vi "FindMaxnIndex.vi"() -> (1 "Numeric":i32, 3 "String":string)   [LabVIEW 2020]
uses:
  <vilib>/Utility/file.llb/Read Delimited Spreadsheet (string).vi
panel:
  out "number":i32[][](array[numeric])
  out "all rows":string[][](array[string])
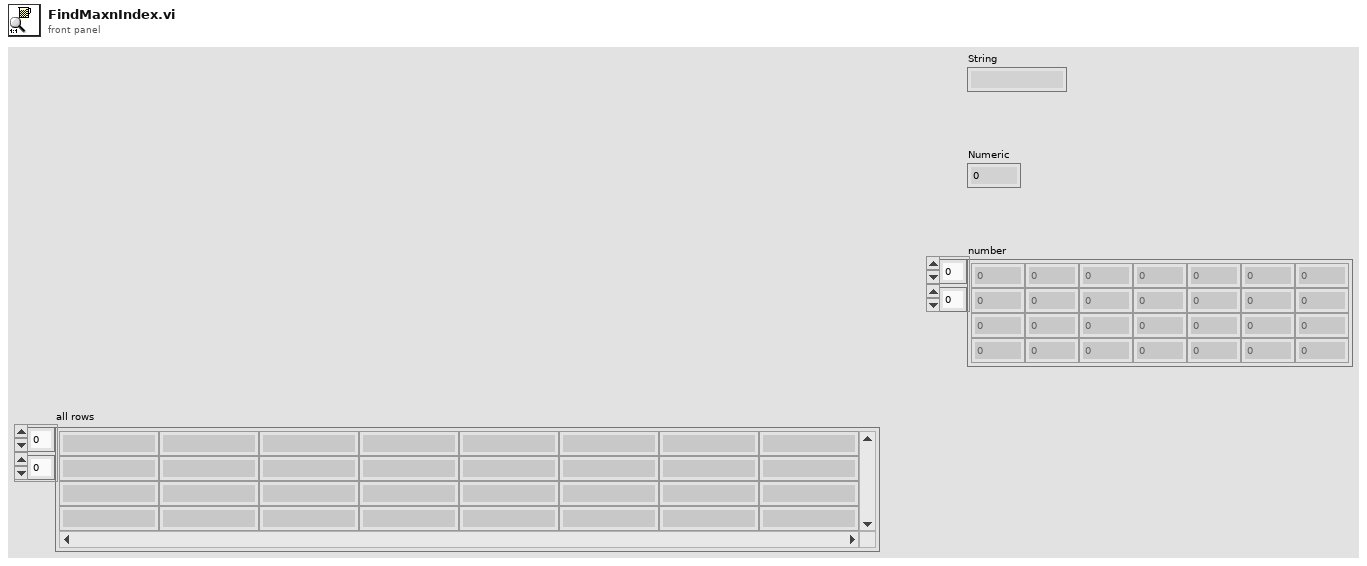
[diagram p1: front panel]
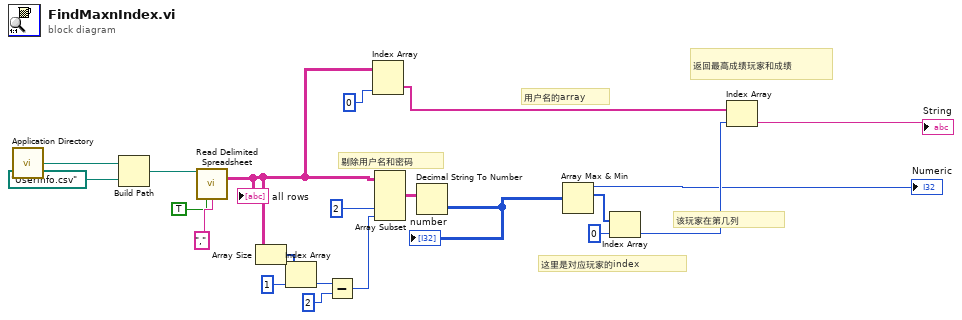
[diagram p0: block diagram]
diagram:
  # "用户名的array"
  # "该玩家在第几列"
  # "返回最高成绩玩家和成绩"
  # "剔除用户名和密码"
  # "这里是对应玩家的index"
  n1 = call <vilib>:"Application Directory.vi"() -> ("Application Directory"=w5:path)
  n2 = Build Path(base path=w5, name or relative path=path "Userinfo.csv") -> (appended path=w1:path)
  n3 = call-poly <vilib>:"Read Delimited Spreadsheet.vi"("file path (dialog if empty)"=w1, "transpose? (F)"=TRUE, "delimiter (\\t)"="," ("delimiter (\\t)")) -> ("all rows"=w17:string[][])  [unwired: 7 in, 5 out]
  "all rows" <- w17
  n4 = Array Size(array=w17) -> (size(s)=w7:i32[])
  n5 = Index Array(array=w7, index=1) -> (element=w9:i32)
  n6 = Subtract(x=w9, y=2 ("index")) -> (x-y=w11:i32)
  n7 = Index Array(array=w17, index (col)=0 ("index (row)")) -> (element=w20:string[])  [unwired: 1 in]
  n8 = Array Subset(array=w17, index (col)=2 ("index"), length (col)=w11) -> (w12:string[][])  [unwired: 2 in]
  n9 = Decimal String To Number(string=w12) -> (number=w14:i32[][])  [unwired: 2 in, 1 out]
  "number" <- w14
  n10 = Array Max & Min(array=w14) -> (max value=→"Numeric":i32, max index (indices)=w16:i32[])  [unwired: 2 out]
  n11 = Index Array(array=w16, index=0) -> (element=w19:i32)
  n12 = Index Array(array=w20, index=w19) -> (element=→"String":string)
